vi "Revision Query.vi"(8 "error in (no error)":errorcluster, 11 "BH Druck PACE Series in":refnum<class "BH Druck PACE Series.lvclass">) -> (0 "error out":errorcluster, 1 "Firmware Revision":string, 2 "Driver Revision":string, 3 "BH Druck PACE Series out":refnum<class "BH Druck PACE Series.lvclass">, 4 "Serial Number":string, 5 "Model":string, 7 "Manufacturer":string)   [LabVIEW 2022 SP3, in "BH Druck PACE Series.lvclass"]
uses:
  BH Druck PACE Series.lvclass
  BH Druck PACE Series.lvclass/BH Druck PACE Series.ctl
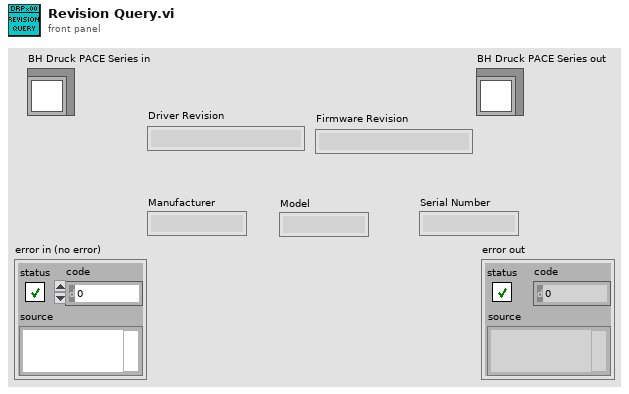
[diagram p1: front panel]
types:
  T1 = cluster{"Major":u16, "Minor":u16, "Fix":u16, "Build":u16}
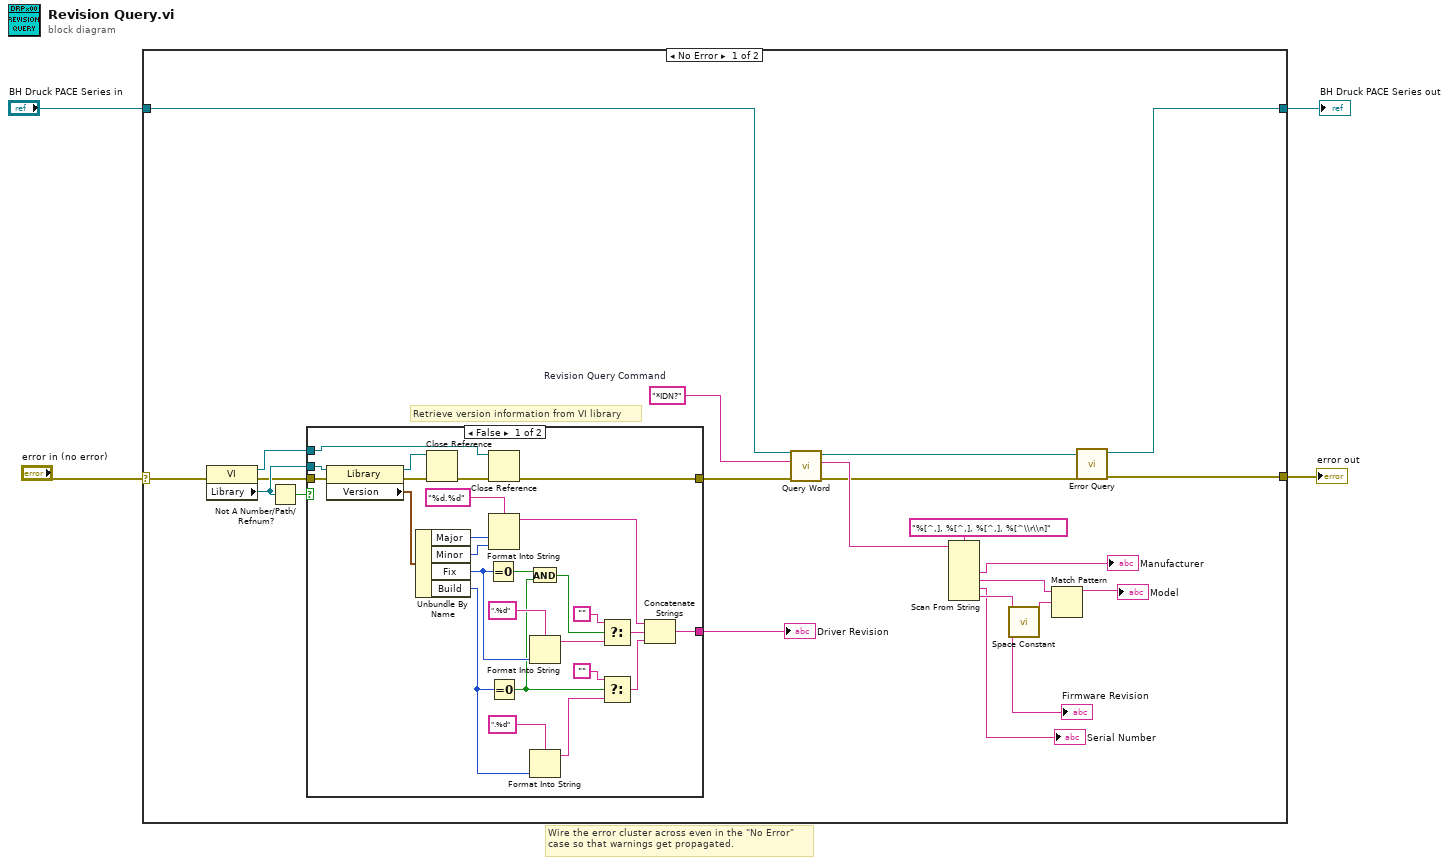
[diagram p0: block diagram]
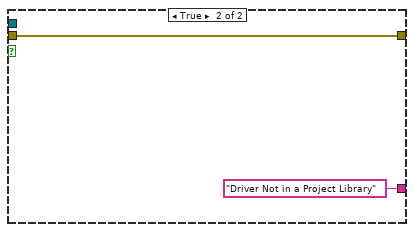
[diagram p2: hidden frame]
diagram:
  # "Wire the error cluster across even in the \"No Error\"\ncase so that warnings get propagated."
  n1 = case shown="No Error" "error in (no error)" {
    selector: "error in (no error)" -> [w21 w55]
    tunnel: [w5 w55] -> w3
    tunnel: [w6 w54] -> w1
    tunnel: "BH Druck PACE Series in" -> [w17 w54]
    frame No Error {
      w18 = "*IDN?"  # Revision Query Command
      # "Retrieve version information from VI library"
      n2 = property on="Property Node" class="VI"(error in=w21) -> (reference out=w22:refnum<vi>, error out=w23:errorcluster, "Library"=w24:refnum<vi>)  [unwired: 1 in]
      n3 = Not A Number/Path/Refnum?(number/path/refnum=w24) -> (NaN/Path/Refnum?=w25:bool)
      n4 = case shown="False" w25 {
        tunnel: w22 -> [w48 _]
        tunnel: w23 -> [w33 w53]
        tunnel: [w28 w53] -> w19
        tunnel: [w27 "Driver Not in a Project Library"] -> w20
        tunnel: w24 -> [w26 _]
        frame False {
          n5 = property on="Property Node" class="Library"(reference=w26, error in=w33) -> (reference out=w50:refnum<vi>, error out=w51:errorcluster, "Version"=w47:T1)
          n6 = Unbundle By Name(w47) -> ("Major"=w36:u16, "Minor"=w35:u16, "Fix"=w32:u16, "Build"=w34:u16)
          n7 = Close Reference(reference=w50, error in (no error)=w51) -> (error out=w49:errorcluster)
          n8 = Equal To 0?(x=w32) -> (x = 0?=w31:bool)
          n9 = Close Reference(reference=w48, error in (no error)=w49) -> (error out=w28:errorcluster)
          n10 = Format Into String(format string="%d.%d", w36, w35) -> (resulting string=w42:string)  [unwired: 2 in, 1 out]
          n11 = Equal To 0?(x=w34) -> (x = 0?=w30:bool)
          n12 = And(x=w31, y=w30) -> (x .and. y?=w29:bool)
          n13 = Format Into String(format string=".%d", w32) -> (resulting string=w44:string)  [unwired: 2 in, 1 out]
          n14 = Format Into String(format string=".%d", w34) -> (resulting string=w40:string)  [unwired: 2 in, 1 out]
          n15 = Select(t="" ("Empty String Constant"), s=w29, f=w44) -> (s? t:f=w41:string)
          n16 = Select(t="" ("Empty String Constant"), s=w30, f=w40) -> (s? t:f=w37:string)
          n17 = Concatenate Strings(w42, w41, w37) -> (w27:string)
        }
        frame True {
        }
      }
      "Driver Revision" <- w20
      n18 = call-dynamic "Query Word.vi"("error in (no error)"=w19, "Query String"=w18, "BH Druck PACE Series in"=w17) -> ("error out"=w8:errorcluster, "String Result"=w9:string, "BH Druck PACE Series out"=w7:refnum<class "BH Druck PACE Series.lvclass">)  [unwired: 6 in]
      n19 = Scan From String(format string="%[^,], %[^,], %[^,], %[^\\r\\n]", input string=w9) -> (output 1=→"Manufacturer":string, output 2=w13:string, output 3=→"Serial Number":string, output 4=→"Firmware Revision":string)  [unwired: 6 in, 3 out]
      n20 = call <vilib>:"Space Constant.vi"() -> ("String"=w14:string)
      n21 = Match Pattern(string=w13, regular expression=w14) -> (before substring=→"Model":string)  [unwired: 1 in, 3 out]
      n22 = call-dynamic "Error Query.vi"("error in (no error)"=w8, "BH Druck PACE Series in"=w7) -> ("error out"=w5:errorcluster, "BH Druck PACE Series out"=w6:refnum<class "BH Druck PACE Series.lvclass">)  [unwired: 8 in]
    }
    frame Error {
    }
  }
  "error out" <- w3
  "BH Druck PACE Series out" <- w1
